vi "ThingWorxResponseErrorCatcher.vi"(8 "error in (no error)":errorcluster, 11 "body":string) -> (0 "error out":errorcluster)   [LabVIEW 2015]
uses:
  <vilib>/regexp/Match Regular Expression.xnode
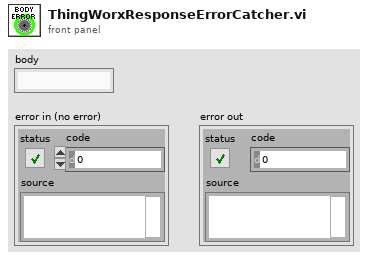
[diagram p1: front panel]
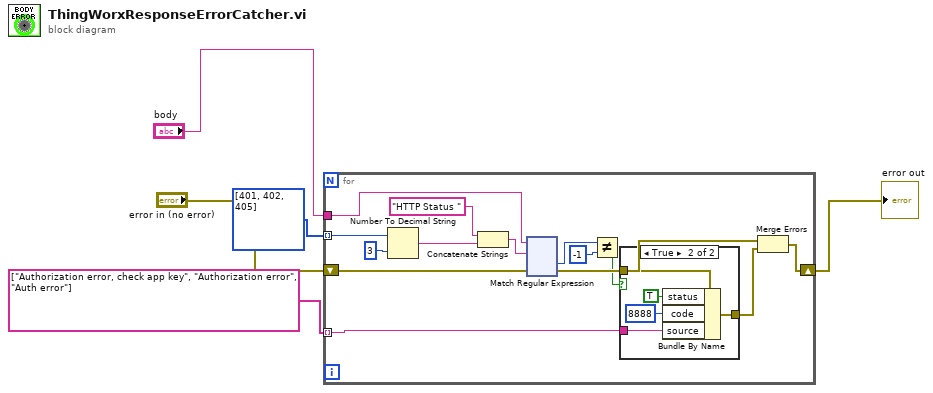
[diagram p0: block diagram]
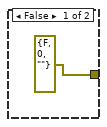
[diagram p2: hidden frame]
diagram:
  n1 = for {
    tunnel: i32[] [401, 402, 405] -> [w16] mode=indexing
    tunnel: "body" -> [w19]
    shift-right: [w10] -> w4
    shift-left: "error in (no error)" -> [w18]
    tunnel: string[] ["Authorization error, check app key", "Authorization error", "Auth error"] -> [w6] mode=indexing
    n2 = Number To Decimal String(number=w16, width (-)=i16 3) -> (decimal integer string=w14:string)
    n3 = Concatenate Strings("HTTP Status ", w14) -> (w13:string)
    n4 = xnode "Match Regular Expression"("input string"=w19, "regular expression"=w13, "error in"=w18) -> ("offset past match"=w12:i32, "error out"=w9:errorcluster)  [unwired: 3 in, 3 out]
    n5 = Not Equal?(x=w12, y=-1) -> (x != y?=w7:bool)
    n6 = case shown="True" w7 {
      tunnel: w9 -> [_ w25]
      tunnel: [errorcluster {"status"=FALSE, "code"=0, "source"=""} ("error constant") w24] -> w8
      tunnel: w6 -> [_ w21]
      frame False {
      }
      frame True {
        n7 = Bundle By Name(cluster=w25, "status"=TRUE, "code"=8888, "source"=w21) -> (w24:errorcluster)
      }
    }
    n8 = Merge Errors(w9, w8) -> (w10:errorcluster)
  }
  "error out" <- w4
